vi "Global Labels.vi"() -> ()   [LabVIEW 2019]
panel:
  out "Labels Array":string[](array[string])
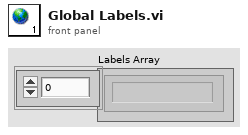
[diagram p1: front panel]
diagram:
